vi "DeleteUser.vi"(3 "error in (no error)":errorcluster, 4 "User_Name":string, 5 "ID":string) -> (0 "error out":errorcluster)   [LabVIEW 2020]
uses:
  <vilib>/Utility/error.llb/DialogType.ctl
  Global_Variable/Global.vi
  <vilib>/addons/database/Connection.llb/DB Tools Open Connec (String).vi
  <vilib>/addons/database/Connection.llb/Conn Execute.vi
  <vilib>/addons/database/Recordset.llb/Rec Destroy - Connection.vi
  <vilib>/addons/database/NI_Database_API.lvlib
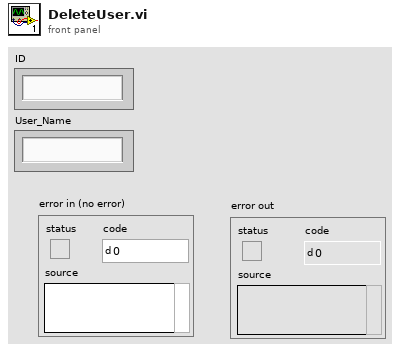
[diagram p1: front panel]
types:
  T1 = typedef "DialogType.ctl" = u16
  T2 = typedef "NI_Database_API.lvlib/Conn ObjectReference.ctl" = refnum<k1>
  T3 = typedef "NI_Database_API.lvlib/Rec ObjectReference.ctl" = refnum<k1>
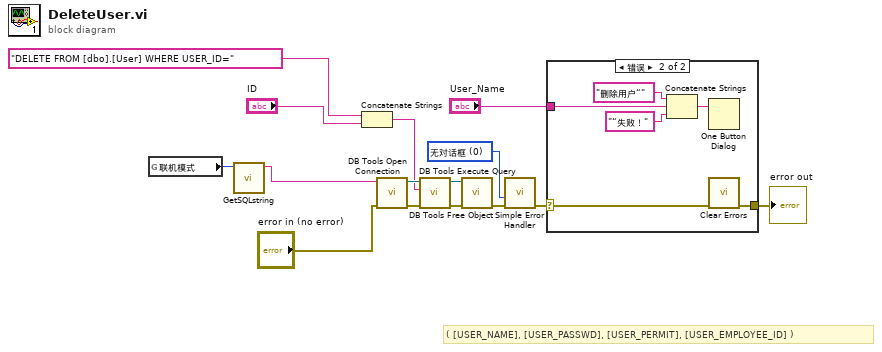
[diagram p0: block diagram]
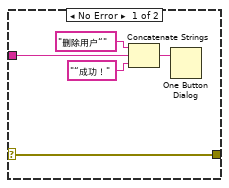
[diagram p2: hidden frame]
diagram:
  w10 = T1 0 items=["无对话框", "确定信息", "继续或停止信息", "确定信息＋警告", "继续/停止+警告"] ("type of dialog (OK msg:1)")
  # "( [USER_NAME], [USER_PASSWD], [USER_PERMIT], [USER_EMPLOYEE_ID] )"
  n1 = global read "Global.vi" "联机模式"() -> (w2:enum16{"单机", "追溯"})
  n2 = call "GetSQLstring.vi"("联机模式"=w2) -> ("连接字符串"=w1:string)  [unwired: 9 in, 1 out]
  n3 = Concatenate Strings("DELETE FROM [dbo].[User] WHERE USER_ID=", "ID") -> (w8:string)
  n4 = call-poly <vilib>:"DB Tools Open Connection.vi"("error in (no error)"="error in (no error)", "connection information"=w1) -> ("error out"=w15:errorcluster, "connection reference"=w14:T2)  [unwired: 6 in]
  n5 = call-poly <vilib>:"DB Tools Execute Query.vi"("error in (no error)"=w15, "SQL query"=w8, "connection reference"=w14) -> ("error out"=w13:errorcluster, "recordset reference"=w12:T3)  [unwired: 5 in]
  n6 = call-poly <vilib>:"DB Tools Free Object.vi"("error in (no error)"=w13, "recordset reference"=w12) -> ("error out"=w11:errorcluster)  [unwired: 8 in, 1 out]
  n7 = call <vilib>:"Simple Error Handler.vi"("type of dialog (OK msg:1)"=w10, "error in (no error)"=w11) -> ("error out"=w4:errorcluster)  [unwired: 3 in, 4 out]
  n8 = case shown="错误" w4 {
    selector: w4 -> [w16 w21]
    tunnel: "User_Name" -> [w17 w23]
    tunnel: [w16 w22] -> w5
    frame No Error {
      n9 = Concatenate Strings("删除用户“" ("消息"), w17, "“成功！" ("消息")) -> (w20:string)
      n10 = One Button Dialog(message=w20) -> ()  [unwired: 1 in, 1 out]
    }
    frame Error {
      n11 = Concatenate Strings("删除用户“" ("消息"), w23, "“失败！" ("消息")) -> (w26:string)
      n12 = One Button Dialog(message=w26) -> ()  [unwired: 1 in, 1 out]
      n13 = call <vilib>:"Clear Errors.vi"("error in (no error)"=w21) -> ("error out"=w22:errorcluster)  [unwired: 5 in, 1 out]
    }
  }
  "error out" <- w5
